vi "EnqueueMessage.vi"(8 "error in (no error)":errorcluster, 9 "Priority":u8, 10 "message":variant, 11 "queue in":refnum<data-value>) -> (0 "error out":errorcluster, 3 "queue out":refnum<data-value>)   [LabVIEW 2013, in "PriorityQueue.lvclass"]
uses:
  PriorityQueue.lvclass
  Message/Message.lvclass
  LinkedList/position.ctl
  LinkedList/InsertSearchOptions.ctl
  PriorityQueue.lvclass/PriorityQueue.ctl
  LinkedList/LinkedList.lvclass
  Common/BasicSortedList/BasicSortedNode/BasicSortedNode.lvclass
  Common/BasicSortedList/BasicSortedList/BasicSortedList.lvclass
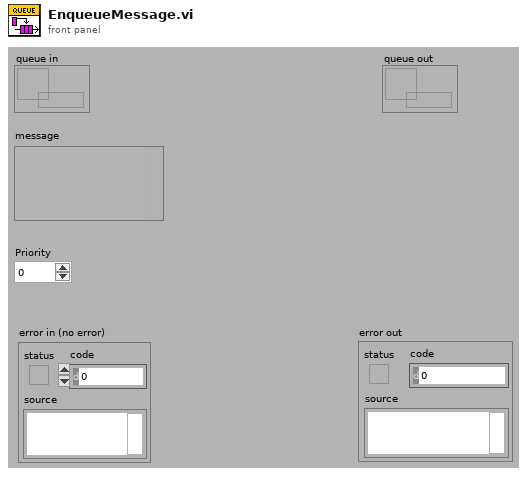
[diagram p1: front panel]
types:
  T1 = typedef "LinkedList.lvclass/InsertSearchOptions.ctl" = cluster{"InsertIfEmpty":bool, "Insert After":bool, "InsertIfNotFound":bool}
  T2 = typedef "LinkedList.lvclass/position.ctl" = enum16{"Front", "Back", "Search"}
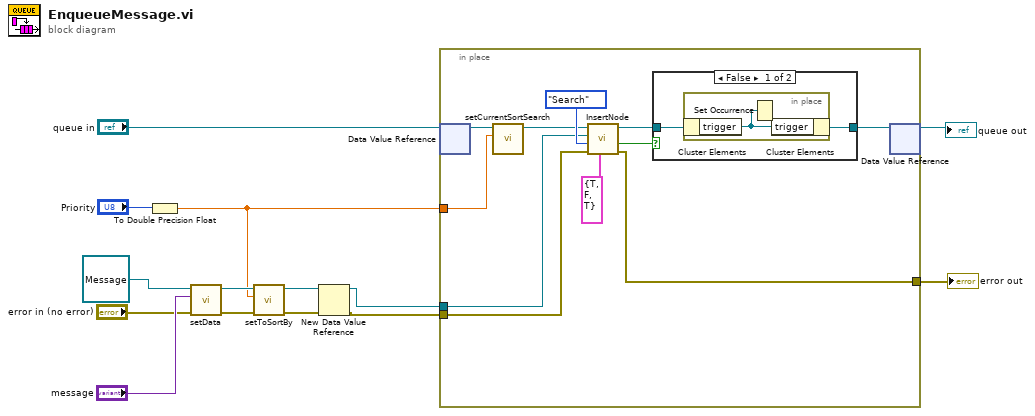
[diagram p0: block diagram]
diagram:
  n1 = To Double Precision Float(number="Priority") -> (double precision float=w5:dbl)
  n2 = call "setData.vi"("error in (no error)"="error in (no error)", "Data"="message", "Message in"=refnum<class "Message.lvclass"> refnum ("Message.lvclass")) -> ("error out"=w7:errorcluster, "Message out"=w8:refnum<class "Message.lvclass">)  [unwired: 7 in]
  n3 = call "setToSortBy.vi"("error in (no error)"=w7, "ToSortBy"=w5, "BasicSortedNode in"=w8) -> ("error out"=w2:errorcluster, "BasicSortedNode out"=w4:refnum<class "Message.lvclass">)  [unwired: 7 in]
  n4 = New Data Value Reference(data value=w4, error in=w2) -> (data value reference=w3:refnum<data-value>, error out=w1:errorcluster)
  n5 = in-place {
    in-place-border: w3 -> [w24]
    in-place-border: w1 -> [w19]
    in-place-border: [w20] -> w12
    in-place-border: w5 -> [w15]
    n6 = in-place-dvr #1("queue in") -> (w17:refnum<class "PriorityQueue.lvclass">)  [unwired: 1 out]
    n7 = call "setCurrentSortSearch.vi"("CurrentSortSearch"=w15, "BasicSortedList in"=w17) -> ("BasicSortedList out"=w16:refnum<class "PriorityQueue.lvclass">)  [unwired: 8 in, 1 out]
    n8 = call "InsertNode.vi"("Insert Search"=T1 {"InsertIfEmpty"=TRUE, "Insert After"=FALSE, "InsertIfNotFound"=TRUE}, "error in (no error)"=w19, "position"=position."Search", "ToInsert"=w24, "LinkedList in"=w16) -> ("error out"=w20:errorcluster, "ignored"=w23:bool, "LinkedList out"=w22:refnum<class "PriorityQueue.lvclass">)  [unwired: 4 in]
    n9 = case shown="False" w23 {
      tunnel: w22 -> [w27 w29]
      tunnel: [w26 w29] -> w21
      frame False {
        n10 = in-place {
          n11 = in-place-cluster #2(w27) -> ("trigger"=w28:refnum<k4>)
          n12 = Set Occurrence(w28) -> ()
          n13 = in-place-cluster #2("trigger"=w28) -> (w26:refnum<class "PriorityQueue.lvclass">)
        }
      }
      frame True {
      }
    }
    n14 = in-place-dvr #1(w21) -> (→"queue out":refnum<data-value>)  [unwired: 1 out]
  }
  "error out" <- w12
